vi "ExternalSetParam.vi"(0 "reference":refnum<class "InterfaceNode.lvclass">, 1 "setParameter":T2, 2 "string":string, 3 "position":T1 {"y" format="%.2f"; "x" format="%.2f"}, 4 "Boolean":bool, 5 "error in (no error)":errorcluster, 7 "ClassPath":path) -> (14 "reference out":refnum<class "InterfaceNode.lvclass">, 19 "error out":errorcluster)   [LabVIEW 2020, in "InterfaceNode.lvclass"]
doc: "Sets parameter externaly.\nPossible to set Name,Attrib,Methods and Position"
uses:
  <resource>/Framework/Providers/Open_GDS/UML/InterfaceNode_class/InterfaceNode.lvclass
  C:/Program Files (x86)/National Instruments/LabVIEW 2020/resource/Framework/Providers/Open_GDS/UML/ClassNode_class/ClassNode.lvclass
  C:/Program Files (x86)/National Instruments/LabVIEW 2020/resource/Framework/Providers/Open_GDS/UML/RectangularNode_class/RectangularNode.lvclass
  <resource>/Framework/Providers/Open_GDS/UML/ClassNode_class/ExternalSetTypes.ctl
  <resource>/Framework/Providers/Open_GDS/UML/General/Point/Point Point2D.ctl
  <resource>/Framework/Providers/Open_GDS/UML/MultiLineString_class/MultiLineString.lvclass
  <resource>/Framework/Providers/Open_GDS/UML/RectangularNode_class/RectangularNode.lvclass
  <resource>/Framework/Providers/Open_GDS/UML/ClassNode_class/ClassNode.lvclass
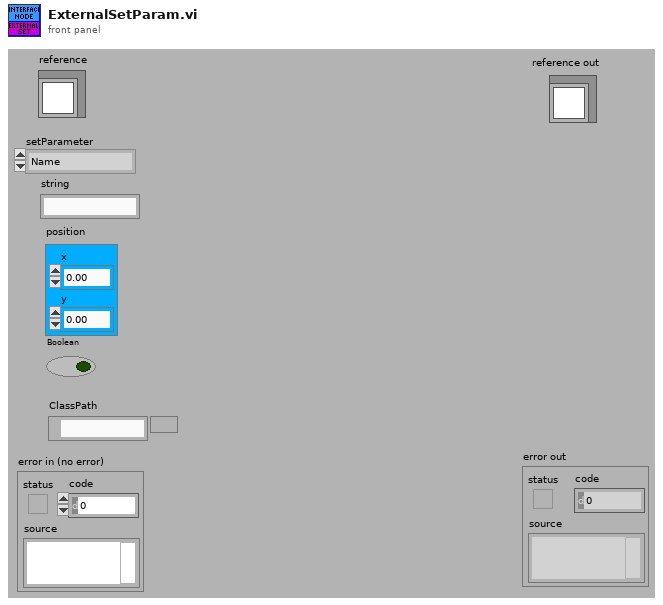
[diagram p1: front panel]
types:
  T1 = typedef "Point Point2D.ctl" = cluster{"x":dbl, "y":dbl}
  T2 = typedef "ClassNode.lvclass/ExternalSetTypes.ctl" = enum16{"Name", "Attributes", "Methods", "Position", "ShowMethods", "ShowAttributes", "ClassPath"}
  T3 = typedef "ClassNode.lvclass/ObjectAttributes.ctl" = cluster{"midHeight":dbl, "botHeight":dbl, "name":refnum<class "MultiLineString.lvclass">, "attributes":refnum<class "MultiLineString.lvclass">, "methods":refnum<class "MultiLineString.lvclass">, "DEFAULT_COMPARTMENT_HEIGHT":i32, "DEFAULT_WIDTH":i32, "DEFAULT_HEIGHT":i32, "showMethods":bool, "showAttributes":bool, "ClassPath":path}
  T4 = typedef "RectangularNode.lvclass/ObjectAttributes.ctl" = cluster{"bounds":T5}
  T5 = typedef "Rectangle Rectangle2D.ctl" = cluster{"x":dbl, "y":dbl, "width":dbl, "height":dbl}
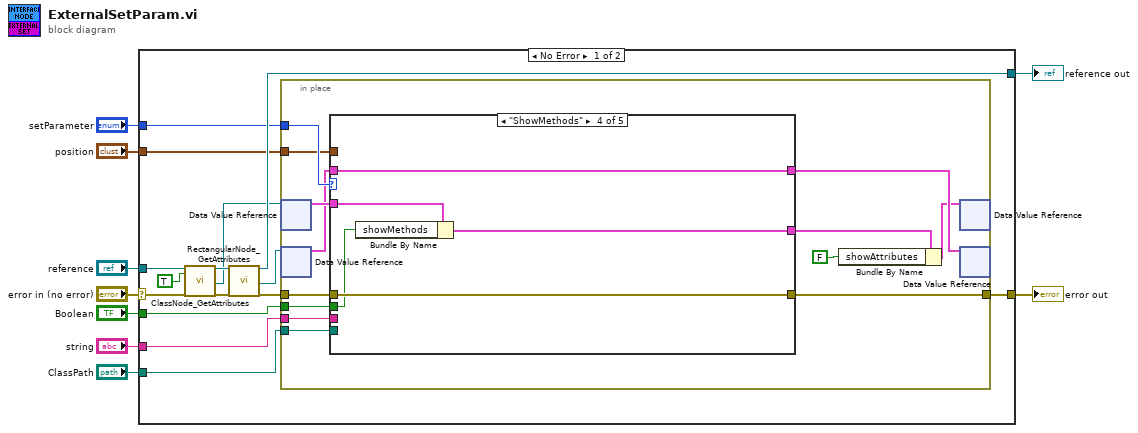
[diagram p0: block diagram]
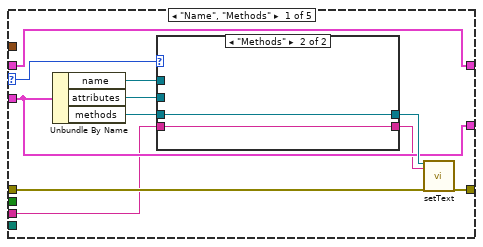
[diagram p2: hidden frame]
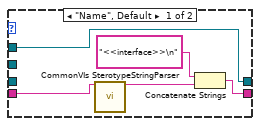
[diagram p3: hidden frame]
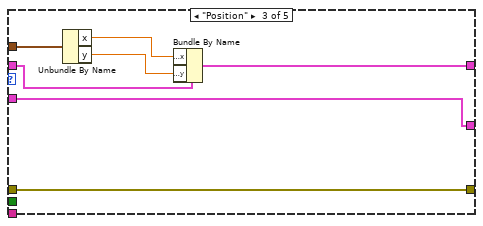
[diagram p5: hidden frame]
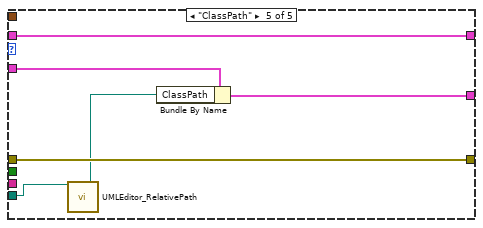
[diagram p6: hidden frame]
diagram:
  n1 = case shown="No Error" "error in (no error)" {
    selector: "error in (no error)" -> [w21 w77]
    tunnel: "reference" -> [w24 w78]
    tunnel: [w23 w77] -> w7
    tunnel: [w22 w78] -> w6
    tunnel: "setParameter" -> [w15 _]
    tunnel: "position" -> [w14 _]
    tunnel: "string" -> [w12 _]
    tunnel: "Boolean" -> [w11 _]
    tunnel: "ClassPath" -> [w10 _]
    frame No Error {
      n2 = call <resource>:"ClassNode_GetAttributes.vi"("reference in"=w24, "OnlyGetDvrReference(False)"=TRUE, "error in (no error)"=w21) -> ("reference out"=w19:refnum<class "InterfaceNode.lvclass">, "DataRef"=w17:refnum<data-value>, "error out"=w18:errorcluster)  [unwired: 13 in, 1 out]
      n3 = call <resource>:"RectangularNode_GetAttributes.vi"("reference in"=w19, "error in (no error)"=w18) -> ("reference out"=w22:refnum<class "InterfaceNode.lvclass">, "DataRef"=w16:refnum<data-value>, "error out"=w13:errorcluster)  [unwired: 14 in, 1 out]
      n4 = in-place {
        in-place-border: w15 -> [w37]
        in-place-border: w14 -> [w36]
        in-place-border: w13 -> [w35]
        in-place-border: w12 -> [w34]
        in-place-border: w11 -> [w33]
        in-place-border: w10 -> [w32]
        in-place-border: [w29] -> w23
        n5 = in-place-dvr #1(w17) -> (w31:T3)  [unwired: 1 out]
        n6 = in-place-dvr #2(w16) -> (w30:T4)  [unwired: 1 out]
        n7 = case shown="\"ShowMethods\"" w37 {
          selector: w37 -> [w48 _ _ _ _]
          tunnel: [w41 w58 w59 w70 w76] -> w26
          tunnel: w36 -> [_ _ w65 _ _]
          tunnel: w35 -> [w47 w56 w62 w69 w75]
          tunnel: [w46 w56 w62 w69 w75] -> w29
          tunnel: w34 -> [w39 _ _ _ _]
          tunnel: w33 -> [_ _ _ w68 _]
          tunnel: w32 -> [_ _ _ _ w73]
          tunnel: w31 -> [w41 w58 w59 w67 w72]
          tunnel: w30 -> [w40 w57 w61 w66 w71]
          tunnel: [w40 w57 w60 w66 w71] -> w28
          frame "Name", "Methods" {
            n8 = Unbundle By Name(w41) -> ("name"=w45:refnum<class "MultiLineString.lvclass">, "attributes"=w43:refnum<class "MultiLineString.lvclass">, "methods"=w42:refnum<class "MultiLineString.lvclass">)
            n9 = case shown="\"Methods\"" w48 {
              tunnel: w45 -> [w53 _]
              tunnel: [w53 w55] -> w44
              tunnel: w43 -> [_ _]
              tunnel: w42 -> [_ w55]
              tunnel: w39 -> [w50 w54]
              tunnel: [w49 w54] -> w38
              frame "Name", Default {
                n10 = call <resource>:"CommonVIs SterotypeStringParser.vi"("SterotypeStringIn"=w50) -> ("Name"=w52:string)  [unwired: 15 in, 3 out]
                n11 = Concatenate Strings("<<interface>>\n" ("text"), w52) -> (w49:string)
              }
              frame "Methods" {
              }
            }
            n12 = call-dynamic "setText.vi"("reference"=w44, "text"=w38, "error in (no error)"=w47) -> ("error out"=w46:errorcluster)  [unwired: 16 out]
          }
          frame Default {
          }
          frame "Position" {
            n13 = Unbundle By Name(w65) -> ("x"=w64:dbl, "y"=w63:dbl)
            n14 = Bundle By Name(cluster=w61, "bounds.x"=w64, "bounds.y"=w63) -> (w60:T4)
          }
          frame "ShowMethods" {
            n15 = Bundle By Name(cluster=w67, "showMethods"=w68) -> (w70:T3)
          }
          frame "ClassPath" {
            n16 = call <resource>:"UMLEditor_RelativePath.vi"("Path In"=w73) -> ("ConvertToRelativePath(If possible)"=w74:path)  [unwired: 1 in, 17 out]
            n17 = Bundle By Name(cluster=w72, "ClassPath"=w74) -> (w76:T3)
          }
        }
        n18 = Bundle By Name(cluster=w26, "showAttributes"=FALSE) -> (w25:T3)
        n19 = in-place-dvr #1(w25) -> ()  [unwired: 2 out]
        n20 = in-place-dvr #2(w28) -> ()  [unwired: 2 out]
      }
    }
    frame Error {
    }
  }
  "reference out" <- w6
  "error out" <- w7
